vi "v0.2_pto_timer_http.vi"(8 "error in":errorcluster, 10 "n pulsos":u32, 11 "mbed.lvclass IN":refnum<class "mbed.lvclass">) -> (0 "error out":errorcluster, 3 "mbed.lvclass OUT":refnum<class "mbed.lvclass">)   [LabVIEW 2011]
doc: "<B>PTO Salida de tren de pulsos</B>\n\nCambiar la frecuencia de salida. Un valor de cero detiene el motor. Existe un valor máximo luego del cual el servomotor se detiene, este valor depende de los paràmetros del driver.\n<B>Frecuencia </B> Valor en hertzios del tren de pulsos a la salida del microcontrolador mbed."
uses:
  C:/mbed/Transport Mechanisms/mbed/mbed.lvclass
  C:/mbed/mbed Interface/RPCFunction/RPCFunction.lvclass
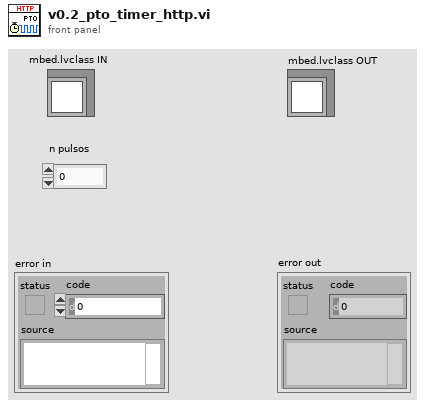
[diagram p1: front panel]
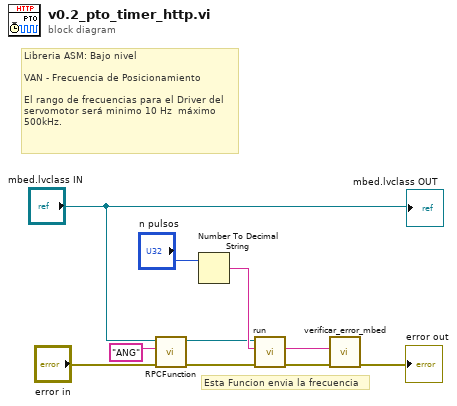
[diagram p0: block diagram]
diagram:
  # "Esta Funcion envia la frecuencia"
  # "Libreria ASM: Bajo nivel          \n\nVAN - Frecuencia de Posicionamiento\n\nEl rango de frecuencias para el Driver del \nservomotor será minimo 10 Hz  máximo\n500kHz."
  n1 = call "RPCFunction.vi"("error in (no error)"="error in", "Existing Obj Name"="ANG", "mbed_LVLibrary.lvlib:mbed.lvclass"="mbed.lvclass IN") -> ("error out"=w4:errorcluster, "mbed_LVLibrary.lvlib:Packet.lvclass 2"=w6:refnum<class "RPCFunction.lvclass">)  [unwired: 6 in, 1 out]
  n2 = Number To Decimal String(number="n pulsos") -> (decimal integer string=w8:string)  [unwired: 1 in]
  n3 = call "run.vi"("error in (no error)"=w4, "Input"=w8, "Packet in"=w6) -> ("error out"=w2:errorcluster, "Output"=w3:string)  [unwired: 6 in, 1 out]
  n4 = call "verificar_error_mbed.vi"("error in (no error)"=w2, "desde_mbed"=w3) -> ("error out"=→"error out":errorcluster)  [unwired: 8 in, 1 out]
  "mbed.lvclass OUT" <- "mbed.lvclass IN"
